vi "AutoSnap DropIn.vi"(8 "error in (no error)":errorcluster, 11 "STOP Notifier":refnum<notifier>) -> (0 "error out":errorcluster)   [LabVIEW 2020]
doc: "This vi should run in parallel with the main loop of its calling vi.\n\nThis vi is used to perform the auto-snap functionality on the calling vi.\n\nPressing F2 (in the calling vi) will lock or unlock the front panel of the calling vi.\n\nWhen locked the user will not be able to move the front panel. If they do it will immediately snap back into position.\n\nWhen unlocked the user can position the vi wherever they like. \n\nCaveats when using this vi.\n1. Before you call this vi, have the fp bounds of the calling vi set to where you want them. The FP must also be open. If you want to the vi to start up without showingf the front panel, you need to use a invoke node to run the FP.Open method and set activate to F and State to Hidden.\n2. This vi runs in its own while loop. Therefore you need to provide a notifier (boolean type ) to tell it when to stop. Simply create a boolean notifier and when the main loop of the calling vi stops, then send a true notification.\n\n\n\nThis vi will cleanup all refnums, including the notifier."
uses:
  <vilib>/event_ctls.llb/eventvkey.ctl
panel:
  # "This vi was written by Sam Taggart.\n\nPlease don't bastardize my code.\nIf you don't understand how it works or need to modify it to suite your application,\nplease contact me.\nIf all else fails, create another copy and bastardize that and leave my pristine copy alone."
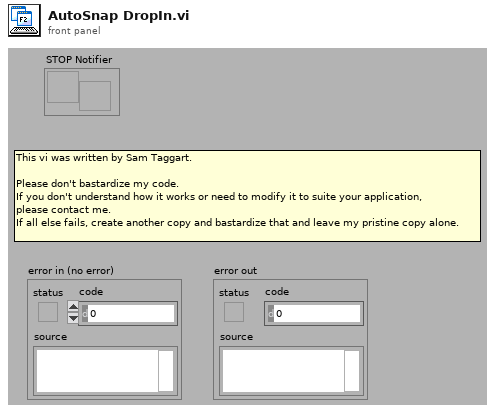
[diagram p1: front panel]
types:
  T1 = typedef "LVRectTypeDef.ctl" = cluster{"Left":i16, "Top":i16, "Right":i16, "Bottom":i16}
  T2 = typedef "LVPointTypeDef.ctl" = cluster{"Horizontal":i16, "Vertical":i16}
  T3 = cluster{"Front Panel.WinBounds":T1, "Front Panel.Origin":T2}
  T4 = typedef "eventvkey.ctl" = enum16{"ASCII", "Enter", "Return", "Shift", "Ctrl", "Alt", "Cmd", "Opt", "Caps", "NumLock", "Clear", "Break", "Up", "Down", "Left", "Right", "Insert", "Delete", "Home", "End", "PageUp", "PageDown", "Escape", "Help", "Pause", "ScrollLock", "F1", "F2", "F3", "F4", "F5", "F6", "F7", "F8", "F9", "F10", "F11", "F12", "F13", "F14", "F15", "F16", "F17", "F18", "F19", "F20", "F21", "F22", "F23", "F24", "Play", "VolumeUp", "VolumeDown", "Mute", "Two Byte Char"}
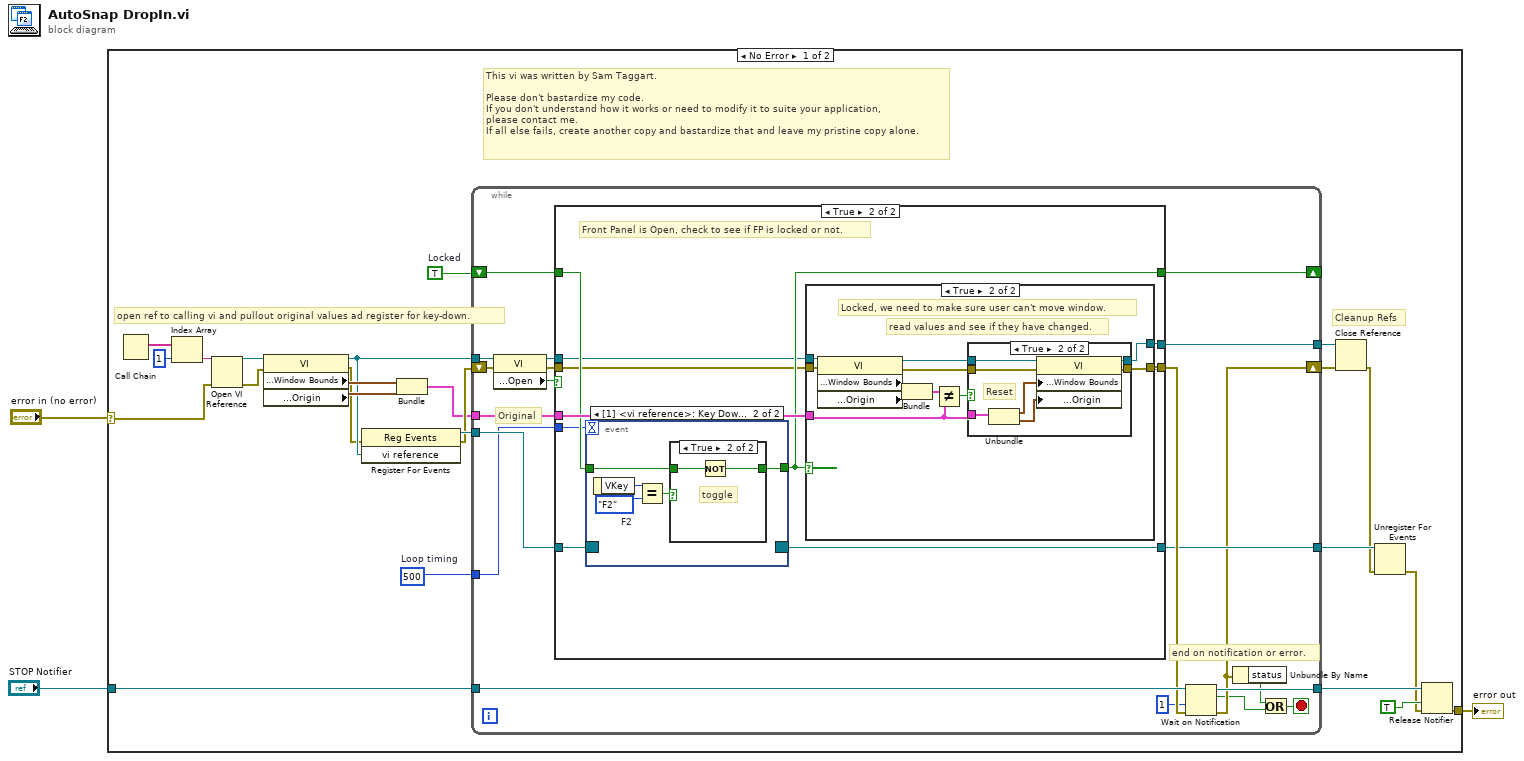
[diagram p0: block diagram]
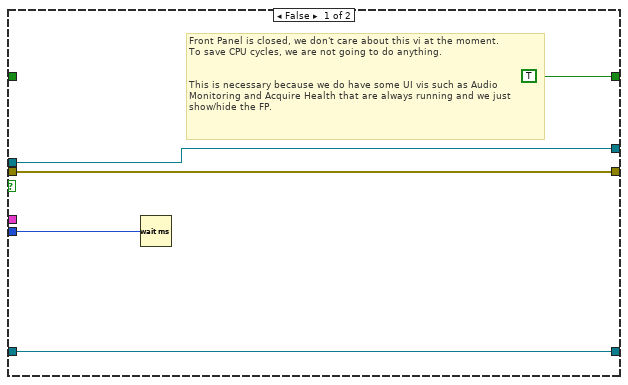
[diagram p2: hidden frame]
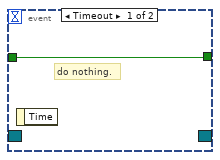
[diagram p5: hidden frame]
diagram:
  n1 = case shown="No Error" "error in (no error)" {
    selector: "error in (no error)" -> [w4 w94]
    tunnel: "STOP Notifier" -> [w20 _]
    tunnel: [w15 w94] -> w2
    frame No Error {
      w5 = 500  # Loop timing
      w13 = TRUE  # Locked
      # "This vi was written by Sam Taggart.\n\nPlease don't bastardize my code.\nIf you don't understand how it works or need to modify it to suite your application,\nplease contact me.\nIf all else fails, create another copy and bastardize that and leave my pristine copy alone."
      # "Cleanup Refs"
      # "open ref to calling vi and pullout original values ad register for key-down."
      n2 = Call Chain() -> (call chain=w27:string[])
      n3 = Index Array(array=w27, index=1) -> (element=w25:string)
      n4 = Open VI Reference(vi path=w25, error in (no error)=w4) -> (vi reference=w24:refnum<vi>, error out=w21:errorcluster)  [unwired: 4 in]
      n5 = property class="VI"(reference=w24, error in=w21) -> (reference out=w14:refnum<vi>, error out=w11:errorcluster, "Front Panel Window:Window Bounds"=w23:T1, "Front Panel Window:Origin"=w22:T2)
      n6 = register-events(error in=w11, w14) -> (reference out=w12:refnum<event-registration>, error out=w10:errorcluster)  [unwired: 1 in]
      n7 = Bundle("Front Panel.WinBounds"=w23, "Front Panel.Origin"=w22) -> (w9:T3)  [unwired: 1 in]
      n8 = while {
        tunnel: w14 -> [w43]
        shift-right: [w33] -> w19
        shift-left: w10 -> [w42]
        tunnel: w20 -> [w47]
        tunnel: [w44] -> w18
        shift-right: [w34] -> _
        shift-left: w13 -> [w35]
        tunnel: [w45] -> w16
        tunnel: w12 -> [w37]
        tunnel: w9 -> [w38]
        tunnel: [w36] -> w8
        tunnel: w5 -> [w29]
        stop <- w30 stop-if-true
        # "end on notification or error."
        # "Original"
        n9 = property class="VI"(reference=w43, error in=w42) -> (reference out=w40:refnum<vi>, error out=w39:errorcluster, "Front Panel.Open"=w41:bool)
        n10 = case shown="True" w41 {
          tunnel: [w52 w62] -> w46
          tunnel: [w50 w61] -> w44
          tunnel: w40 -> [w50 w55]
          tunnel: w39 -> [w52 w54]
          tunnel: w38 -> [_ w60]
          tunnel: w37 -> [w51 w59]
          tunnel: [w51 w58] -> w36
          tunnel: w35 -> [_ w57]
          tunnel: [TRUE ("Locked") w56] -> w34
          tunnel: w29 -> [w48 w53]
          frame False {
            # "Front Panel is closed, we don't care about this vi at the moment.\nTo save CPU cycles, we are not going to do anything.\n\n\nThis is necessary because we do have some UI vis such as Audio\nMonitoring and Acquire Health that are always running and we just\nshow/hide the FP."
            n11 = Wait (ms)(milliseconds to wait=w48) -> ()  [unwired: 1 out]
          }
          frame True {
            # "Front Panel is Open, check to see if FP is locked or not."
            n12 = event shown="[1] <vi reference>: Key Down" {
              selector: w59 -> [_ _]
              dyn-events: [_ _] -> w58
              timeout: w53 -> [_ _]
              tunnel: w57 -> [w85 w87]
              tunnel: [w85 w86] -> w56
              event Timeout {
                # "do nothing."
                n13 = event-data() -> ()  [unwired: 1 in, 1 out]
              }
              event Key Down {
                w89 = eventvkey."F2"  # F2
                n14 = event-data() -> ("VKey"=w90:T4)  [unwired: 1 in]
                n15 = Equal?(x=w90, y=w89) -> (x = y?=w88:bool)
                n16 = case shown="True" w88 {
                  tunnel: w87 -> [w91 w93]
                  tunnel: [w91 w92] -> w86
                  frame False {
                    # "do nothing."
                  }
                  frame True {
                    # "toggle"
                    n17 = Not(x=w93) -> (.not. x?=w92:bool)
                  }
                }
              }
            }
            n18 = case shown="True" w56 {
              tunnel: [w64 w70] -> w62
              tunnel: [w63 w68] -> w61
              tunnel: w60 -> [_ w67]
              tunnel: w55 -> [w63 w66]
              tunnel: w54 -> [w64 w65]
              frame False {
                # "Unlocked, user can move window wherever they like.\nWe need to do nothing."
              }
              frame True {
                # "Locked, we need to make sure user can't move window."
                # "read values and see if they have changed."
                n19 = property class="VI"(reference=w66, error in=w65) -> (reference out=w69:refnum<vi>, error out=w71:errorcluster, "Front Panel Window:Window Bounds"=w75:T1, "Front Panel Window:Origin"=w74:T2)
                n20 = Bundle("Front Panel.WinBounds"=w75, "Front Panel.Origin"=w74) -> (w73:T3)  [unwired: 1 in]
                n21 = Not Equal?(x=w73, y=w67) -> (x != y?=w72:bool)
                n22 = case shown="True" w72 {
                  tunnel: w71 -> [w77 w82]
                  tunnel: [w77 w81] -> w70
                  tunnel: w67 -> [_ w80]
                  tunnel: w69 -> [w76 w84]
                  tunnel: [w76 w83] -> w68
                  frame False {
                    # "no change - do nothing."
                  }
                  frame True {
                    # "Reset"
                    n23 = Unbundle(w80) -> ("Front Panel.WinBounds"=w79:T1, "Front Panel.Origin"=w78:T2)
                    n24 = property class="VI"(reference=w84, error in=w82, "Front Panel Window:Window Bounds"=w79, "Front Panel Window:Origin"=w78) -> (reference out=w83:refnum<vi>, error out=w81:errorcluster)
                  }
                }
              }
            }
          }
        }
        n25 = Wait on Notification(notifier=w47, timeout in ms (-1)=1, error in (no error)=w46) -> (notifier out=w45:refnum<notifier>, notification=w31:bool, error out=w33:errorcluster)  [unwired: 1 in, 1 out]
        n26 = Unbundle By Name(w33) -> ("status"=w32:bool)
        n27 = Or(x=w32, y=w31) -> (x .or. y?=w30:bool)
      }
      n28 = Close Reference(reference=w18, error in (no error)=w19) -> (error out=w7:errorcluster)
      n29 = Unregister For Events(event registration refnum=w8, error in=w7) -> (error out=w6:errorcluster)
      n30 = Release Notifier(notifier=w16, force destroy? (F)=TRUE, error in (no error)=w6) -> (error out=w15:errorcluster)  [unwired: 2 out]
    }
    frame Error {
    }
  }
  "error out" <- w2
